vi "Set Tx Generic Session.vi"(8 "error in":errorcluster, 9 "Redundant?":bool, 10 "session_tx_generic":T2[](array[typedef]) {"StartMode" items=["FDX_STOP", "FDX_START", "FDX_START_TRG", "FDX_START_TIME"]}, 11 "Ports Ref":T1 format="%.0x") -> (0 "error out":errorcluster, 3 "Ports Ref Out":T1 format="%.0x")   [LabVIEW 2020, in "AIM ARINC 664 Scripting.lvlib"]
uses:
  AIM ARINC 664 Scripting.lvlib
  Shared/session_tx_generic.ctl
  Import/AIM ARINC 664 Import.lvlib
  <vilib>/NI VeriStand/Custom Device API/Custom Device Item Ref.ctl
  <vilib>/NI VeriStand/Custom Device API/Custom Device API.lvlib
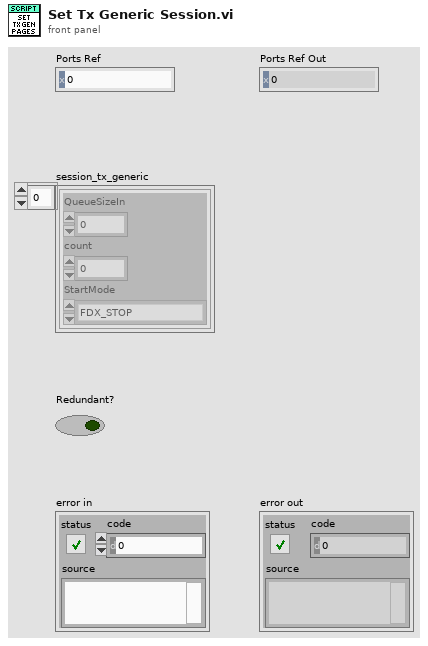
[diagram p1: front panel]
types:
  T1 = typedef "Custom Device API.lvlib/Custom Device Item Ref.ctl" = u64
  T2 = typedef "AIM ARINC 664 Import.lvlib/session_tx_generic.ctl" = cluster{"QueueSizeIn":u32, "count":i32, "StartMode":i32}
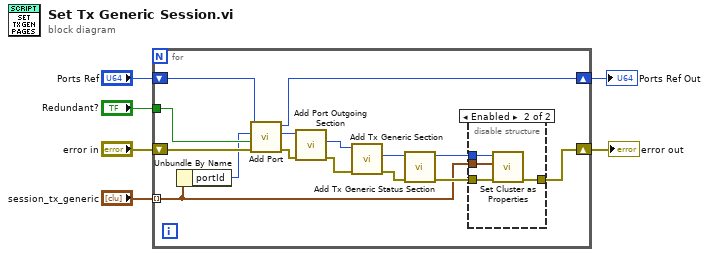
[diagram p0: block diagram]
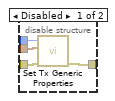
[diagram p2: hidden frame]
diagram:
  n1 = for {
    tunnel: "session_tx_generic" -> [w8] mode=indexing
    shift-right: [w21] -> w5
    shift-left: "error in" -> [w17]
    tunnel: "Redundant?" -> [w9]
    shift-right: [w10] -> w1
    shift-left: "Ports Ref" -> [w14]
    n2 = Unbundle By Name(w8) -> ("portId"=w7:u32)
    n3 = call "Add Port.vi"("error in"=w17, "Redundant"=w9, "portId"=w7, "Ports Ref"=w14) -> ("error out"=w15:errorcluster, "Port Ref out"=w11:T1, "Parent Ref out"=w10:T1)  [unwired: 5 in]
    n4 = call "Add Port Outgoing Section.vi"("error in"=w15, "Port Ref"=w11) -> ("error out"=w16:errorcluster, "Port Outgoing Ref out"=w19:T1)  [unwired: 7 in, 1 out]
    n5 = call "Add Tx Generic Section.vi"("error in"=w16, "Port Outgoing Ref"=w19) -> ("error out"=w18:errorcluster, "Section Ptr"=w13:T1)  [unwired: 7 in, 1 out]
    n6 = call "Add Tx Generic Status Section.vi"("error in"=w18, "Section Ref in"=w13) -> ("error out"=w20:errorcluster, "Section Ref out"=w12:T1)  [unwired: 6 in, 2 out]
    n7 = disable-structure shown="Enabled" {
      disable-tunnel: [w25 w28] -> w21
      disable-tunnel: w20 -> [w24 w29]
      disable-tunnel: w8 -> [w23 w27]
      disable-tunnel: w12 -> [w22 w26]
      frame Disabled {
        n8 = call "Set Tx Generic Properties.vi"("error in"=w24, "session_tx_generic"=w23, "custom device ref in"=w22) -> ("error out"=w25:errorcluster)  [unwired: 7 in, 1 out]
      }
      frame Enabled {
        n9 = call "Set Cluster as Properties.vi"("error in"=w29, "Variant Cluster"=w27, "custom device ref in"=w26) -> ("error out"=w28:errorcluster)  [unwired: 7 in, 1 out]
      }
    }
  }
  "error out" <- w5
  "Ports Ref Out" <- w1
